vi "Read Waveform.vi"   [LabVIEW 2021, in "Siglent SDS 1000 2000 Series.lvlib"]
doc: "This VI select the type of read: Single Waveform or Multiple Waveform."
uses:
  <instrlib>/Siglent SDS 1000 2000 Series/Siglent SDS 1000 2000 Series.lvlib
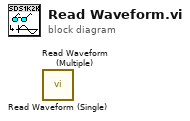
[diagram p0: block diagram]
diagram:
  n1 = call <instrlib>:"Read Waveform (Single).vi"() -> ()  [unwired: 9 in, 3 out]
  n2 = call <instrlib>:"Read Waveform (Multiple).vi"() -> ()  [unwired: 9 in, 3 out]
